vi "Flip Frame.vi"(9 "Flip Vertically":bool, 10 "Flip Horizontally":bool, 11 "Input Array":u16[][](array[numeric])) -> (3 "output array":u16[][](array[numeric]))   [LabVIEW 2023, in "Camera.lvlib"]
uses:
  Camera.lvlib
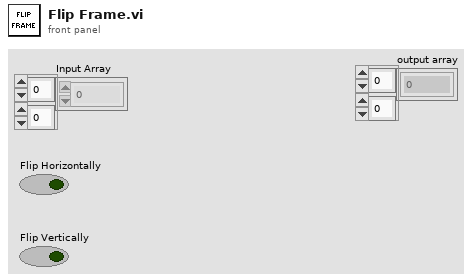
[diagram p1: front panel]
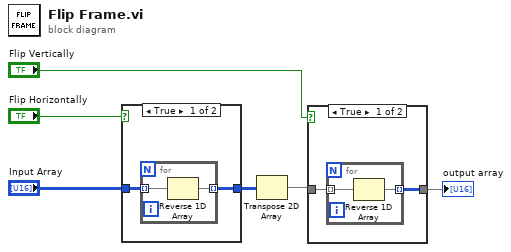
[diagram p0: block diagram]
diagram:
  n1 = case shown="True" "Flip Horizontally" {
    tunnel: "Input Array" -> [w7 w11]
    tunnel: [w8 w11] -> w5
    frame True {
      n2 = for {
        tunnel: w7 -> [w10] mode=indexing
        tunnel: [w9] -> w8 mode=indexing
        n3 = Reverse 1D Array(array=w10) -> (reversed array=w9:u16[])
      }
    }
    frame False {
    }
  }
  n4 = Transpose 2D Array(2D array=w5) -> (transposed array=w4:u16[][])
  n5 = case shown="True" "Flip Vertically" {
    tunnel: w4 -> [w12 w16]
    tunnel: [w13 w16] -> w3
    frame True {
      n6 = for {
        tunnel: w12 -> [w15] mode=indexing
        tunnel: [w14] -> w13 mode=indexing
        n7 = Reverse 1D Array(array=w15) -> (reversed array=w14:u16[])
      }
    }
    frame False {
    }
  }
  "output array" <- w3
